vi "Event Test.vi"(8 "error in (no error)":errorcluster, 11 "user event out":refnum<user-event>) -> (0 "error out":errorcluster)   [LabVIEW 2014]
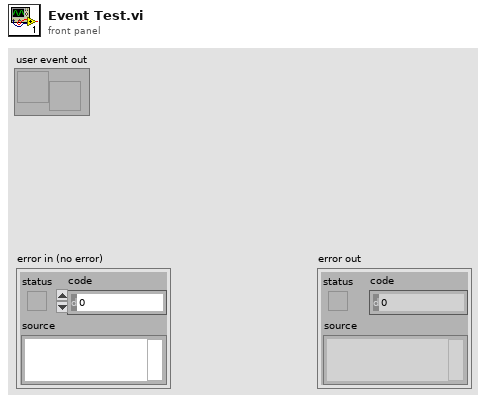
[diagram p1: front panel]
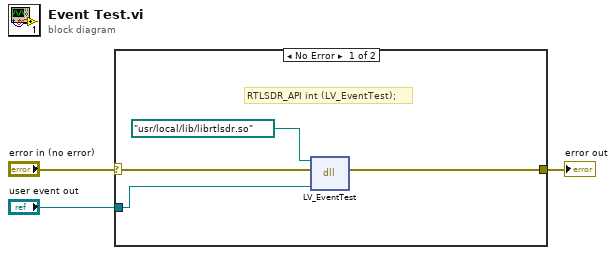
[diagram p0: block diagram]
diagram:
  n1 = case shown="No Error" "error in (no error)" {
    selector: "error in (no error)" -> [w5 w8]
    tunnel: [w7 w8] -> w3
    tunnel: "user event out" -> [w4 _]
    frame No Error {
      # "RTLSDR_API int (LV_EventTest);"
      n2 = dll-call lib="usr/local/lib/librtlsdr.so" fn="LV_EventTest"(path in=path "/usr/local/lib/librtlsdr.so", error in=w5, "msg"=w4) -> (error out=w7:errorcluster)  [unwired: 3 in, 1 out]
    }
    frame Error {
    }
  }
  "error out" <- w3
